vi "Interface initialize.vi"(8 "error in":errorcluster, 11 "TCP interface in":refnum<class "TCP Interface.lvclass">) -> (0 "error out":errorcluster, 3 "TCP interface out":refnum<class "TCP Interface.lvclass">)   [LabVIEW 2021, in "TCP Interface.lvclass"]
doc: "Opens a TCP connection to the address and port stored in the class."
uses:
  TCP Interface.lvclass
  TCP Interface.lvclass/TCP Interface.ctl
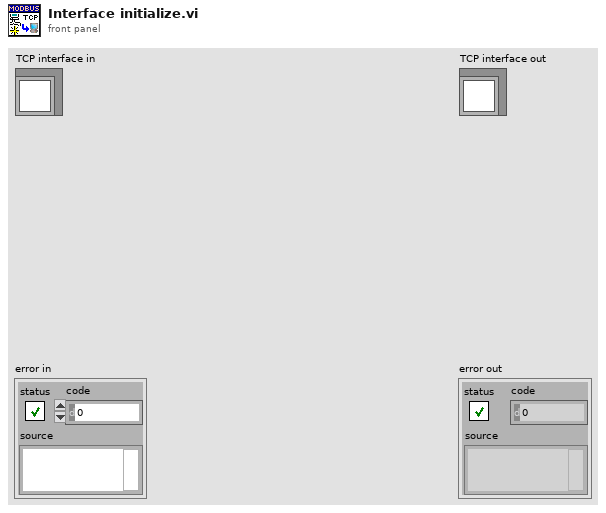
[diagram p1: front panel]
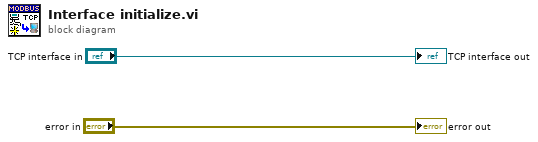
[diagram p0: block diagram]
diagram:
  "error out" <- "error in"
  "TCP interface out" <- "TCP interface in"
